vi "get Contact wfm.vi"(0 "reference in":refnum<class "Force Curve_tdms.lvclass">, 5 "error in (no error)":errorcluster) -> (14 "reference out":refnum<class "Force Curve_tdms.lvclass">, 16 "Samples contact out":i32, 19 "error out":errorcluster)   [LabVIEW 2019, in "Force Curve_tdms.lvclass"]
uses:
  Force Curve_tdms.lvclass
  private/Signal In.ctl
  <vilib>/Waveform/WDTOps.llb/WDT Get Waveform Subset DBL.vi
panel:
  in  "t":dbl=3.0 format="%#_13g"
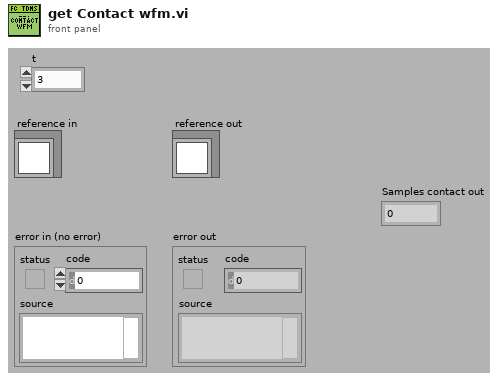
[diagram p1: front panel]
types:
  T1 = typedef "Force Curve_tdms.lvclass/Signal In.ctl" = enum16{"Deflection", "SensorIn", "MockOut", "ZstageOut"}
  T2 = typedef "Force Curve_tdms.lvclass/ObjectAttributesRef.ctl" = refnum<data-value>
  T3 = typedef "Force Curve_tdms.lvclass/ObjectAttributes.ctl" = cluster{"MyAttribute":dbl, "Processed data":waveform(dbl)[], "Fcurve Raw Metadata":T4, "Fcurve Metadata":T5, "Fcurve index":T6, "Tau Delay (ms)":dbl, "Contact Spread of dev":dbl, "Fcurve":T7}
  T4 = typedef "TDMS_DataHandler.lvclass/Fcurve Meta data.ctl" = cluster{"property names":string[], "property values":variant[]}
  T5 = typedef "Force Curve_tdms.lvclass/Fcurve Meta data analysis.ctl" = cluster{"dt (us)":dbl, "Dec Factor":dbl, "Z piezo Sensitivity (nm/V)":dbl, "K (N/m)":dbl, "Sp (V)":dbl, "Contact (ms)":dbl, "Zpos contact":dbl, "Vel_app (nm/s)":dbl, "Vel_ret (nm/s)":dbl, "deltaV (nm)":dbl, "Def_V0 (v)":dbl, "Decimating Factor":dbl}
  T6 = typedef "Force Curve_tdms.lvclass/Fcurve Index .ctl" = cluster{"Setpoint index":i32, "Max force index":i32, "Contact point index":i32, "Appoach indices":cluster{"Start":i32, "End":i32}, "Contact indices":cluster{"Start":i32, "End":i32}, "Retract indices":cluster{"Start":i32, "End":i32}}
  T7 = typedef "Force Curve_tdms.lvclass/Force Curve data.ctl" = cluster{"Approach":cluster{"X":dbl[], "Y":dbl[]}, "Contact":cluster{"X":dbl[], "Y":dbl[]}, "Retract":cluster{"X":dbl[], "Y":dbl[]}}
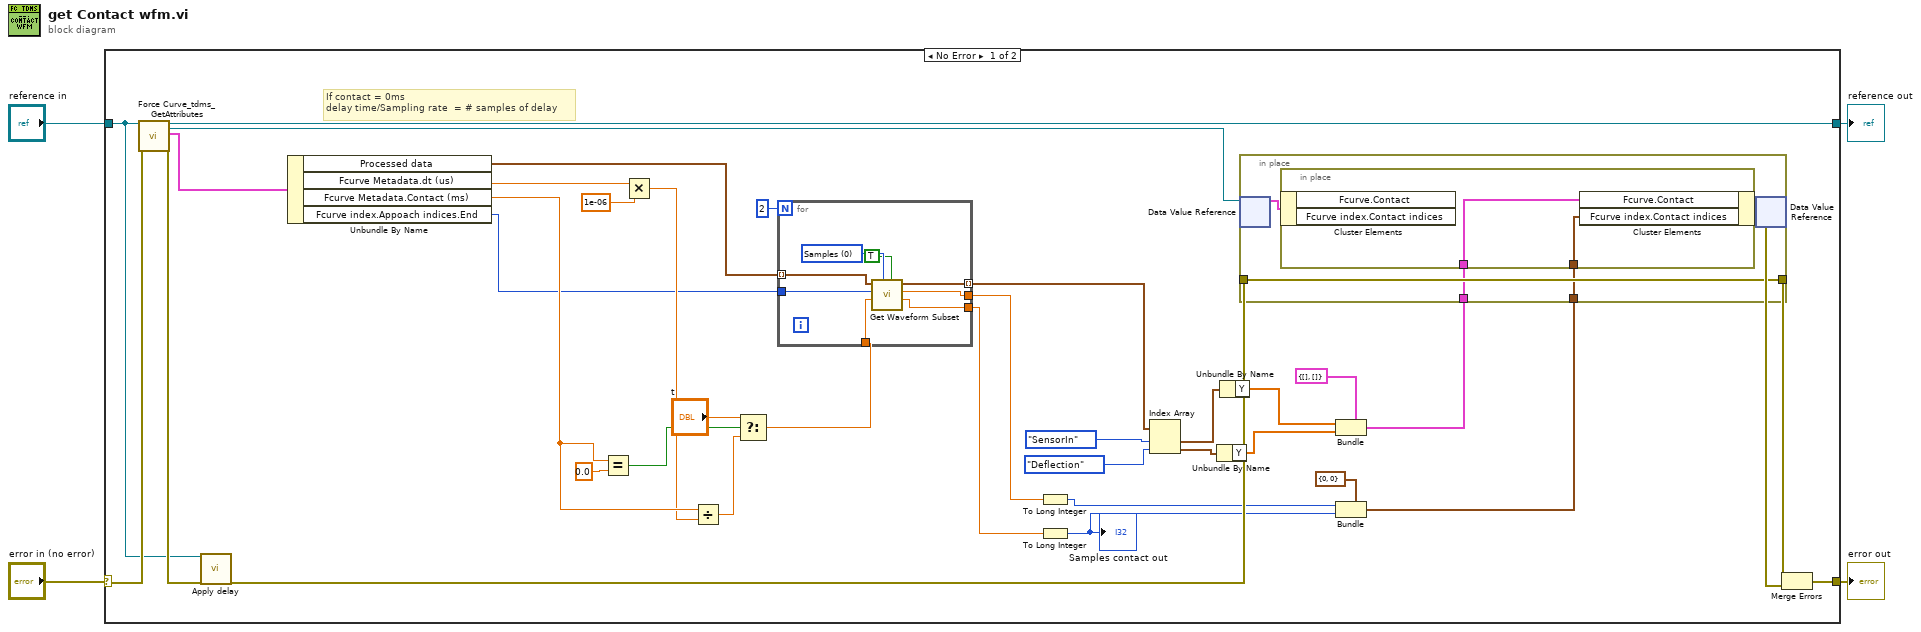
[diagram p0: block diagram]
diagram:
  n1 = case shown="No Error" "error in (no error)" {
    selector: "error in (no error)" -> [w39 w58]
    tunnel: [w41 w58] -> w3
    tunnel: [w40 w57] -> w1
    tunnel: "reference in" -> [w31 w57]
    frame No Error {
      # "If contact = 0ms\ndelay time/Sampling rate  = # samples of delay"
      n2 = call "Force Curve_tdms_GetAttributes.vi"("reference in"=w31, "error in (no error)"=w39) -> ("reference out"=w40:refnum<class "Force Curve_tdms.lvclass">, "attributes ref"=w35:T2, "attributes"=w38:T3, "error out"=w33:errorcluster)  [unwired: 14 in]
      n3 = call "Apply delay.vi"("reference in"=w31, "error in (no error)"=w33) -> ("error out"=w32:errorcluster)  [unwired: 15 in, 2 out]
      n4 = Unbundle By Name(w38) -> ("Processed data"=w34:waveform(dbl)[], "Fcurve Metadata.dt (us)"=w21:dbl, "Fcurve Metadata.Contact (ms)"=w16:dbl, "Fcurve index.Appoach indices.End"=w11:i32)
      n5 = Equal?(x=w16, y=0.0) -> (x = y?=w17:bool)
      n6 = Multiply(x=w21, y=1e-06) -> (x*y=w15:dbl)
      n7 = Divide(x=w16, y=w15) -> (x/y=w13:dbl)
      n8 = Select(t="t", s=w17, f=w13) -> (s? t:f=w14:dbl)
      n9 = for {
        N: 2 -> [_]
        tunnel: [w48] -> w12
        tunnel: [w47] -> w28 mode=indexing
        tunnel: w34 -> [w46] mode=indexing
        tunnel: w11 -> [w42]
        tunnel: w14 -> [w45]
        tunnel: [w43] -> w7
        w49 = u16 0 items=["Samples", "Relative Time"] ("start/duration format")
        n10 = call-poly <vilib>:"Get Waveform Subset.vi"("open interval? (T)"=TRUE, "start/duration format"=w49, "duration"=w45, "start samples/time"=w42, "waveform in"=w46) -> ("actual duration"=w48:dbl, "actual start samples/time"=w43:dbl, "waveform out"=w47:waveform(dbl))  [unwired: 1 in, 1 out]
      }
      n11 = To Long Integer(number=w7) -> (32bit integer=w6:i32)
      n12 = To Long Integer(number=w12) -> (32bit integer=w8:i32)
      "Samples contact out" <- w8
      n13 = Index Array(array=w28, index #1=Signal_In."SensorIn" ("Signal in"), index #2=Signal_In."Deflection" ("Signal in")) -> (element #1=w25:waveform(dbl), element #2=w24:waveform(dbl))
      n14 = Unbundle By Name(w24) -> ("Y"=w23:dbl[])
      n15 = Unbundle By Name(w25) -> ("Y"=w22:dbl[])
      n16 = Bundle(cluster=cluster{"X":dbl[], "Y":dbl[]} {"X"=[], "Y"=[]} ("Fcurve.Approach"), "X"=w22, "Y"=w23) -> (w29:cluster{"X":dbl[], "Y":dbl[]})
      n17 = Bundle(cluster=cluster{"Start":i32, "End":i32} {"Start"=0, "End"=0} ("Fcurve index.Contact indices"), "Start"=w6, "End"=w8) -> (w9:cluster{"Start":i32, "End":i32})
      n18 = in-place {
        in-place-border: w32 -> [w52]
        in-place-border: [w52] -> w37
        in-place-border: w29 -> [w51]
        in-place-border: w9 -> [w50]
        n19 = in-place-dvr #1(w35) -> (w53:T3)  [unwired: 1 out]
        n20 = in-place {
          in-place-border: w51 -> [w56]
          in-place-border: w50 -> [w55]
          n21 = in-place-cluster #2(w53) -> ()  [unwired: 2 out]
          n22 = in-place-cluster #2("Fcurve.Contact"=w56, "Fcurve index.Contact indices"=w55) -> (w54:T3)
        }
        n23 = in-place-dvr #1(w54) -> (w36:errorcluster)  [unwired: 1 out]
      }
      n24 = Merge Errors(w37, w36) -> (w41:errorcluster)
    }
    frame Error {
    }
  }
  "error out" <- w3
  "reference out" <- w1
